vi "getSize.vi"(0 "reference":refnum<class "MultiLineString.lvclass">, 5 "error in (no error)":errorcluster) -> (14 "reference out":refnum<class "MultiLineString.lvclass">, 15 "size":T1, 19 "error out":errorcluster)   [LabVIEW 2016, in "MultiLineString.lvclass"]
doc: "public int getSize()"
uses:
  <resource>/Framework/Providers/Open_GDS/UML/MultiLineString_class/MultiLineString.lvclass
  <resource>/Framework/Providers/Open_GDS/UML/MultiLineString_class/SizeType.ctl
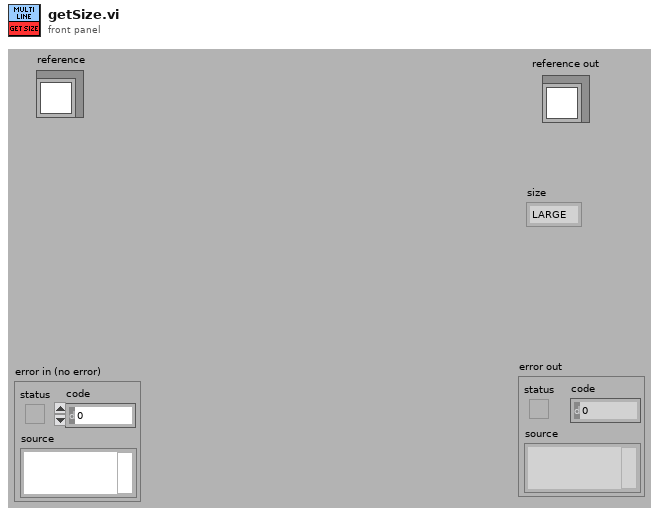
[diagram p1: front panel]
types:
  T1 = typedef "MultiLineString.lvclass/SizeType.ctl" = enum16{"LARGE", "NORMAL", "SMALL"}
  T2 = typedef "MultiLineString.lvclass/ObjectAttributes.ctl" = cluster{"GAP":i32, "text":string, "justification":T3, "size":T1, "underlined":bool}
  T3 = typedef "MultiLineString.lvclass/JustificationType.ctl" = enum16{"LEFT", "CENTER", "RIGHT"}
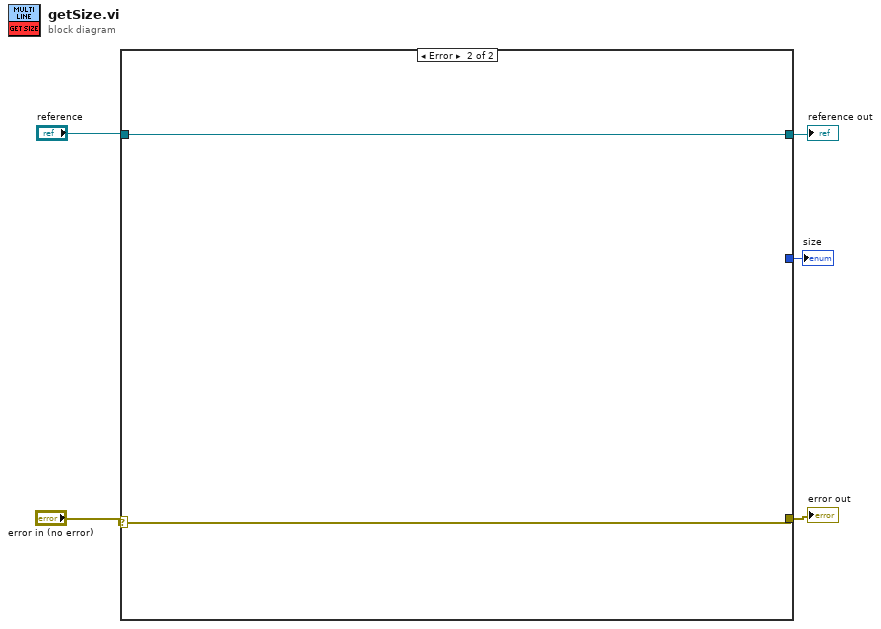
[diagram p0: block diagram]
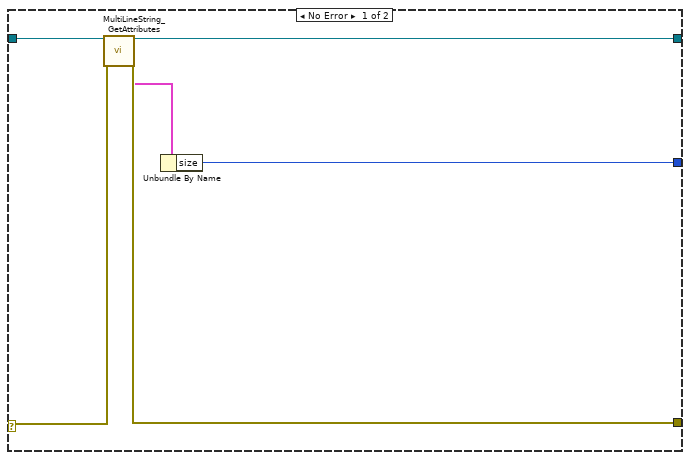
[diagram p2: hidden frame]
diagram:
  n1 = case shown="Error" "error in (no error)" {
    selector: "error in (no error)" -> [w8 w12]
    tunnel: "reference" -> [w11 w13]
    tunnel: [w10 w12] -> w3
    tunnel: [w9 w13] -> w2
    tunnel: [w7 _] -> w1
    frame No Error {
      n2 = call <resource>:"MultiLineString_GetAttributes.vi"("reference in"=w11, "error in (no error)"=w8) -> ("reference out"=w9:refnum<class "MultiLineString.lvclass">, "Data"=w6:T2, "error out"=w10:errorcluster)  [unwired: 1 in, 14 out]
      n3 = Unbundle By Name(w6) -> ("size"=w7:T1)
    }
    frame Error {
    }
  }
  "reference out" <- w2
  "error out" <- w3
  "size" <- w1
